vi "Update database.vi"(8 "error in (no error)":errorcluster, 10 "Name":string, 11 "Paquetes Disponibles in":refnum<class "Paquetes Disponibles.lvclass">) -> (0 "error out":errorcluster, 3 "Paquetes Disponibles out":refnum<class "Paquetes Disponibles.lvclass">)   [LabVIEW 2020, in "Paquetes Disponibles.lvlib" / "Paquetes Disponibles.lvclass"]
uses:
  Paquetes Disponibles.lvclass
  Paquetes Disponibles.lvclass/Paquetes Disponibles.ctl
  <vilib>/drjdpowell/SQLite Library/SQL Connection/Open (path).vi
  <vilib>/drjdpowell/SQLite Library/SQL Connection/Open (string).vi
  <vilib>/AdvancedString/Path To Command Line String.vi
  <vilib>/drjdpowell/SQLite Library/SQL Connection/Execute SQL (No results).vi
  <vilib>/drjdpowell/SQLite Library/SQL Connection/Connection.lvclass
  <vilib>/drjdpowell/SQLite Library/SQLite.lvlib
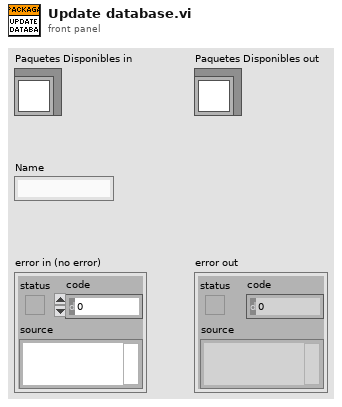
[diagram p1: front panel]
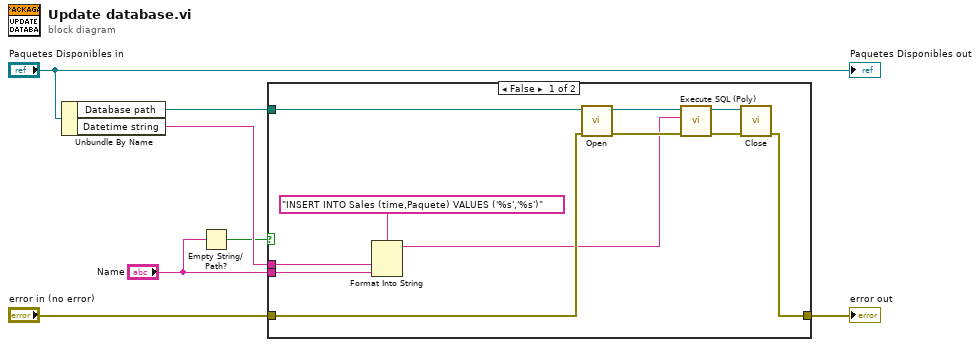
[diagram p0: block diagram]
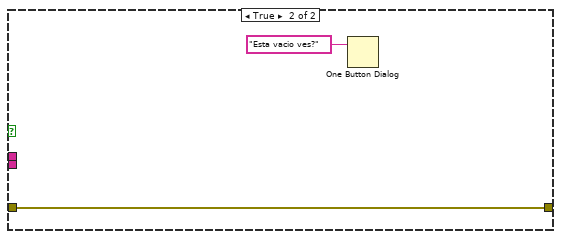
[diagram p2: hidden frame]
diagram:
  n1 = Unbundle By Name("Paquetes Disponibles in") -> ("Database path"=w6:path, "Datetime string"=w3:string)
  n2 = Empty String/Path?(string/path="Name") -> (empty?=w1:bool)
  n3 = case shown="False" w1 {
    tunnel: w6 -> [w18 _]
    tunnel: "error in (no error)" -> [w15 w19]
    tunnel: [w14 w19] -> w4
    tunnel: w3 -> [w9 _]
    tunnel: "Name" -> [w8 _]
    frame False {
      n4 = Format Into String(format string="INSERT INTO Sales (time,Paquete) VALUES ('%s','%s')", w9, w8) -> (resulting string=w11:string)  [unwired: 2 in, 1 out]
      n5 = call-poly <vilib>:"Open.vi"("error in (no error)"=w15, "db file"=w18) -> ("error out"=w12:errorcluster, "SQLite Connection"=w17:refnum<class "Connection.lvclass">)  [unwired: 8 in]
      n6 = call-poly <vilib>:"Execute SQL (Poly).vi"("error in (no error)"=w12, "SQL"=w11, "SQLite Connection in"=w17) -> ("error out"=w13:errorcluster, "SQLite Connection"=w16:refnum<class "Connection.lvclass">)  [unwired: 7 in]
      n7 = call-dynamic "Close.vi"("error in (no error)"=w13, "SQLite Connection in"=w16) -> ("error out"=w14:errorcluster)  [unwired: 9 in]
    }
    frame True {
      n8 = One Button Dialog(message="Esta vacio ves?") -> ()  [unwired: 1 in, 1 out]
    }
  }
  "error out" <- w4
  "Paquetes Disponibles out" <- "Paquetes Disponibles in"
